vi "Read configuration.vi"(7 "force loading?":bool=TRUE, 8 "error in (no error)":errorcluster, 11 "Thorcam in":refnum<class "Thorcam.lvclass">) -> (0 "error out":errorcluster, 3 "Thorcam out":refnum<class "Thorcam.lvclass">)   [LabVIEW 2012, in "Thorcam.lvclass"]
doc: "Reads the XML-based configuration file and populates the configuration cluster accordingly. Configuration file name is <component ID>.xml."
uses:
  Thorcam.lvclass
  <vilib>/Distrio/Murmex/Murmex/Murmex.lvclass
  Thorcam.lvclass/Thorcam.ctl
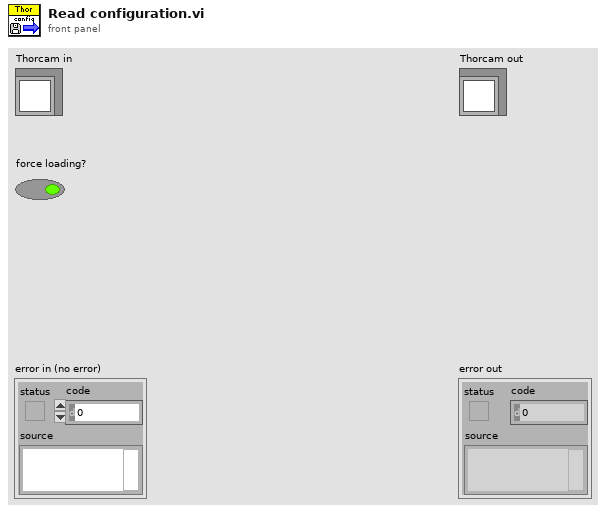
[diagram p1: front panel]
types:
  T1 = typedef "Thorcam.lvclass/configuration.ctl" = cluster{"camera ID1":u32, "Settings":string, "Cross Correlation method":T2, "Reporting folder":path, "LUT":path, "Stage component":string, "Background image":path, "camera ID2":u32, "select camera":u32, "Shift to defocus conversion factor":dbl, "Alignment quality threshold":dbl}
  T2 = typedef "Thorcam.lvclass/cross correlation method.ctl" = enum16{"default", "normalised cross correlation", "normalised mutual information", "binary cross correlation"}
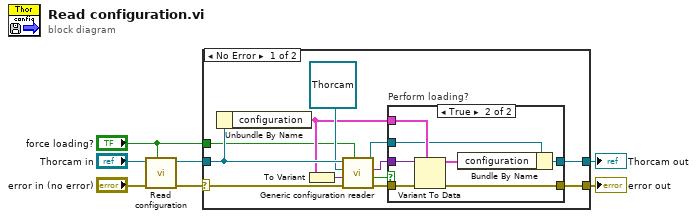
[diagram p0: block diagram]
diagram:
  n1 = call-parent "Read configuration.vi"("force loading?"="force loading?", "error in (no error)"="error in (no error)", "Murmex in"="Thorcam in") -> ("error out"=w5:errorcluster, "Murmex out"=w3:refnum<class "Thorcam.lvclass">)  [unwired: 7 in]
  n2 = case shown="No Error" w5 {
    selector: w5 -> [w18 w30]
    tunnel: [w16 w30] -> w4
    tunnel: w3 -> [w15 w29]
    tunnel: [w11 w29] -> w2
    tunnel: "force loading?" -> [w8 _]
    frame No Error {
      n3 = Unbundle By Name(w15) -> ("configuration"=w13:T1)
      n4 = To Variant(anything=w13) -> (Variant=w19:variant)
      n5 = call <vilib>:"Generic configuration reader.vi"("force loading?"=w8, "error in (no error)"=w18, "configuration cluster variant"=w19, "inheritance level"=refnum<class "Thorcam.lvclass"> refnum ("Thorcam"), "Murmex in"=w15) -> ("error out"=w17:errorcluster, "loaded?"=w10:bool, "configuration data (variant)"=w9:variant, "Murmex out"=w12:refnum<class "Thorcam.lvclass">)  [unwired: 3 in]
      n6 = case "Perform loading?" shown="True" w10 {
        tunnel: [w20 w25] -> w11
        tunnel: [w21 w28] -> w16
        tunnel: w17 -> [w21 w26]
        tunnel: w13 -> [_ w24]
        tunnel: w12 -> [w20 w23]
        tunnel: w9 -> [_ w22]
        frame False {
        }
        frame True {
          n7 = Variant To Data(error in=w26, type=w24, Variant=w22) -> (data=w27:T1, error out=w28:errorcluster)
          n8 = Bundle By Name(cluster=w23, "configuration"=w27) -> (w25:refnum<class "Thorcam.lvclass">)
        }
      }
    }
    frame Error {
    }
  }
  "error out" <- w4
  "Thorcam out" <- w2
